vi "test2.vi"() -> ()   [LabVIEW 2014]
uses:
  <userlib>/ROS for LabVIEW Software/ROS/Code/Console/Servers/ServerSubs/TopicDef.ctl
  <userlib>/ROS for LabVIEW Software/ROS/Code/SubVIs/_ROSDirection.ctl
  <userlib>/ROS for LabVIEW Software/ROS/Code/_ROSDefinition.vi
  <userlib>/ROS for LabVIEW Software/ROS/MessageBuilding/std_msgs/subs/stringScalar.vi
  <userlib>/ROS for LabVIEW Software/ROS/MessageBuilding/std_msgs/subs/float32Scalar.vi
  <userlib>/ROS for LabVIEW Software/ROS/MessageBuilding/std_msgs/subs/i32Scalar.vi
panel:
  in  "Array":i32[](array[numeric])
  in  "ROS Master":string="172.16.0.10:11311"
  in  "Numeric":sgl
  in  "I said:":string="Hello world!"
  out "error out":errorcluster
  in  "stop":bool
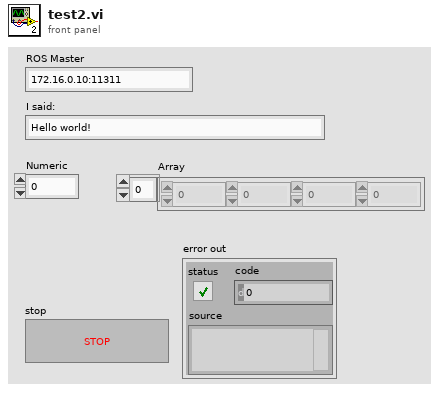
[diagram p1: front panel]
types:
  T1 = typedef "TopicDef.ctl" = cluster{"Topic":string, "Type":string, "Action":T2, "Update (ms)":u16, "queue size":u16}
  T2 = typedef "_ROSDirection.ctl" = enum16{"Node", "Publisher", "Subscriber", "ServiceClient", "ServiceProvider"}
  T3 = typedef "_ROSControl.ctl" = cluster{"topic port":u16, "Node":string, "topic":string, "type":string, "node port":u16, "error ":errorcluster, "Direction":T2, "Update (ms)":u16, "FIFO size":u16}
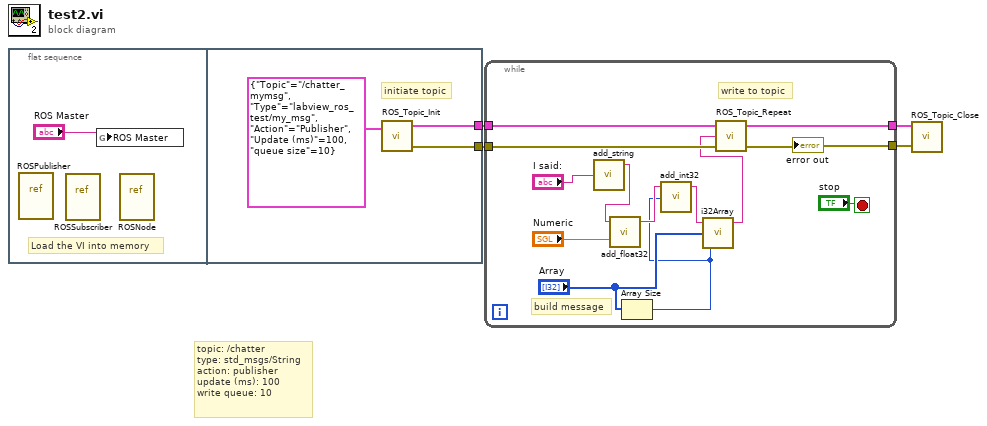
[diagram p0: block diagram]
diagram:
  # "topic: /chatter\ntype: std_msgs/String\naction: publisher\nupdate (ms): 100\nwrite queue: 10"
  n1 = flat-sequence {
    tunnel: [w7] -> w4
    tunnel: [w6] -> w3
    frame #0 {
      # "Load the VI into memory"
      n2 = vi-ref <userlib>:"ROSPublisher.vi"() -> ()  [unwired: 1 out]
      n3 = vi-ref <userlib>:"ROSSubscriber.vi"() -> ()  [unwired: 1 out]
      n4 = global write "_ROSDefinition.vi" "ROS Master"("ROS Master") -> ()
      n5 = vi-ref <userlib>:"ROSNode.vi"() -> ()  [unwired: 1 out]
    }
    frame #1 {
      # "initiate topic"
      n6 = call <userlib>:"ROS_Topic_Init.vi"("Definitions"=T1 {"Topic"="/chatter_mymsg", "Type"="labview_ros_test/my_msg", "Action"=enum."Publisher", "Update (ms)"=100, "queue size"=10}) -> ("ROS out"=w7:T3, "error out"=w6:errorcluster)  [unwired: 2 in]
    }
  }
  n7 = while {
    tunnel: w4 -> [w21]
    tunnel: w3 -> [w19]
    tunnel: [w17] -> w2
    tunnel: [w16] -> w1
    stop <- "stop" stop-if-true
    # "build message"
    # "write to topic"
    n8 = call-poly <userlib>:"add_string.vi"("String"="I said:") -> ("msg out"=w14:string)  [unwired: 4 in]
    n9 = call-poly <userlib>:"add_float32.vi"("Numeric"="Numeric", "msg in"=w14) -> ("msg out"=w11:string)  [unwired: 3 in]
    n10 = Array Size(array="Array") -> (size(s)=w9:i32)
    n11 = call-poly <userlib>:"add_int32.vi"("Numeric"=w9, "msg in"=w11) -> ("msg out"=w10:string)  [unwired: 3 in]
    n12 = call <userlib>:"i32Array.vi"("Array Length"=w9, "Array"="Array", "msg in"=w10) -> ("msg out"=w13:string)  [unwired: 2 in]
    n13 = call <userlib>:"ROS_Topic_Repeat.vi"("error in (no error)"=w19, "Msg in"=w13, "ROS in"=w21) -> ("error out"=w16:errorcluster, "ROS out"=w17:T3)  [unwired: 1 in]
    "error out" <- w16
  }
  n14 = call <userlib>:"ROS_Topic_Close.vi"("error in"=w1, "ROS in"=w2) -> ()  [unwired: 2 in, 1 out]
